vi "Create.vi"(8 "error in (no error)":errorcluster, 10 "Barcode Content":string) -> (0 "error out":errorcluster, 3 "Barcode Reader Out":refnum<class "Barcode.lvclass">)   [LabVIEW 2020, in "Barcode Reader Second Iteration.lvlib" / "Barcode.lvclass"]
uses:
  Barcode.lvclass
  Type A/Type A.lvclass
  C:/Git/astemes-gdevcon-2022/Barcode Reader Demo/Barcode Reader Second Iteration/Barcode Reader/Barcode Reader.lvclass
  Type B/Type B.lvclass
  Barcode.lvclass/Barcode.ctl
  C:/Git/astemes-gdevcon-2022/Barcode Reader Demo/Barcode Reader Second Iteration/Barcode Reader/Barcode.lvclass
  C:/Git/astemes-gdevcon-2022/Barcode Reader Demo/Barcode Reader Second Iteration/Type A/Type A.lvclass
  C:/Git/astemes-gdevcon-2022/Barcode Reader Demo/Barcode Reader Second Iteration/Type B/Type B.lvclass
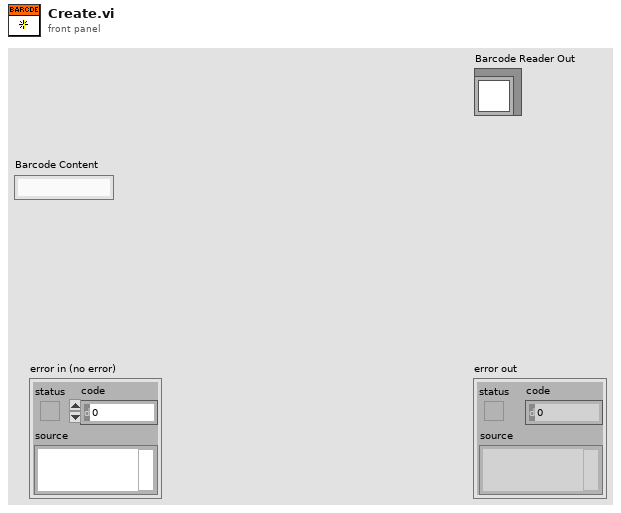
[diagram p1: front panel]
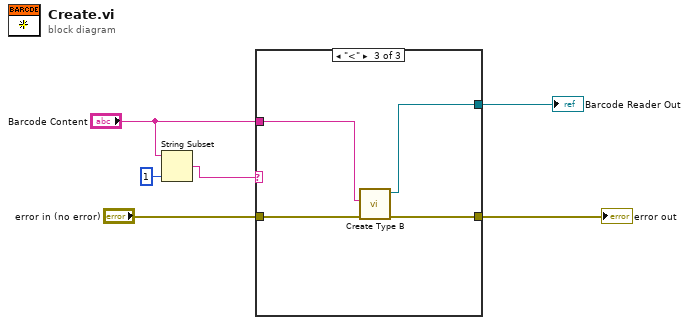
[diagram p0: block diagram]
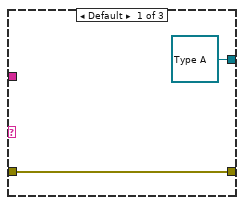
[diagram p2: hidden frame]
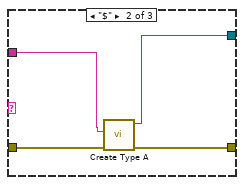
[diagram p3: hidden frame]
diagram:
  n1 = String Subset(string="Barcode Content", length (rest)=1 ("length (rest)")) -> (substring=w1:string)  [unwired: 1 in]
  n2 = case shown="\"<\"" w1 {
    tunnel: "error in (no error)" -> [w7 w12 w15]
    tunnel: [w7 w11 w14] -> w5
    tunnel: [refnum<class "Type A.lvclass"> refnum ("Barcode Reader out") w10 w13] -> w4
    tunnel: "Barcode Content" -> [_ w9 w16]
    frame Default {
    }
    frame "$" {
      n3 = call "Create Type A.vi"("error in (no error)"=w12, "Barcode Content"=w9) -> ("error out"=w11:errorcluster, "Barcode Reader out"=w10:refnum<class "Type A.lvclass">)  [unwired: 8 in]
    }
    frame "<" {
      n4 = call "Create Type B.vi"("error in (no error)"=w15, "Barcode Content"=w16) -> ("error out"=w14:errorcluster, "Barcode Reader out"=w13:refnum<class "Type B.lvclass">)  [unwired: 8 in]
    }
  }
  "error out" <- w5
  "Barcode Reader Out" <- w4
